vi "ROI entry-Event handler-Arb entry.vi"(8 "error in (no error)":errorcluster) -> (0 "error out":errorcluster)   [LabVIEW 2013]
uses:
  Typedefs/ROI ID Enum.ctl
  ROI Entry screen/Globals/gl_ROI Entry UI globals.vi
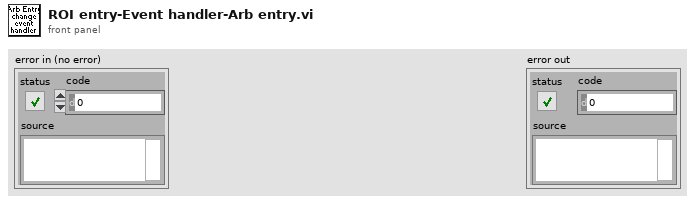
[diagram p1: front panel]
types:
  T1 = typedef "ROI entry screen ctrl refs cluster.ctl" = cluster{"Done button":refnum<vi>, "Imaging button":refnum<vi>, "Acquisition button":refnum<vi>, "POI dwell time (us)":refnum<vi>, "Scan dwell time per pixel (us)":refnum<vi>, "# of planes":refnum<vi>, "Zoom":refnum<vi>, "Equal size":refnum<vi>, "Channel":refnum<vi>, "Image Display":refnum<vi>, "Z-Plane Selector":refnum<vi>, "Number of lines left":refnum<vi>, "Z-stack folder path":refnum<vi>, "POI Density":refnum<vi>, "Arb Plane Entry":refnum<vi>, "Whole plane":refnum<vi>, "Clear Last":refnum<vi>, "Clear All":refnum<vi>, "Trial Length (sec)":refnum<vi>, "Palette Type":refnum<vi>, "Intensity slider":refnum<vi>, "# POI":refnum<vi>, "Max Z Proj":refnum<vi>, "Zplane ind":refnum<vi>, "Wavelength (nm)":refnum<vi>, "Number of Trials":refnum<vi>, "Funct stim.trig.enable":refnum<vi>, "Funct stim.trig.delay (s)":refnum<vi>, "Line Mode":refnum<vi>, "Step size (µm)":refnum<vi>, "ROI move mode":refnum<vi>, "Cool-down time (s)":refnum<vi>, "Enable cool-down time":refnum<vi>, "Motor Z ind. (um)":refnum<vi>, "AOL Z ind. (um)":refnum<vi>}
  T2 = typedef "ROI ID Enum.ctl" = enum16{"Point", "MiniScan", "Comp. MiniScan", "Rectangle", "Comp. volume", "Arb. plane point"}
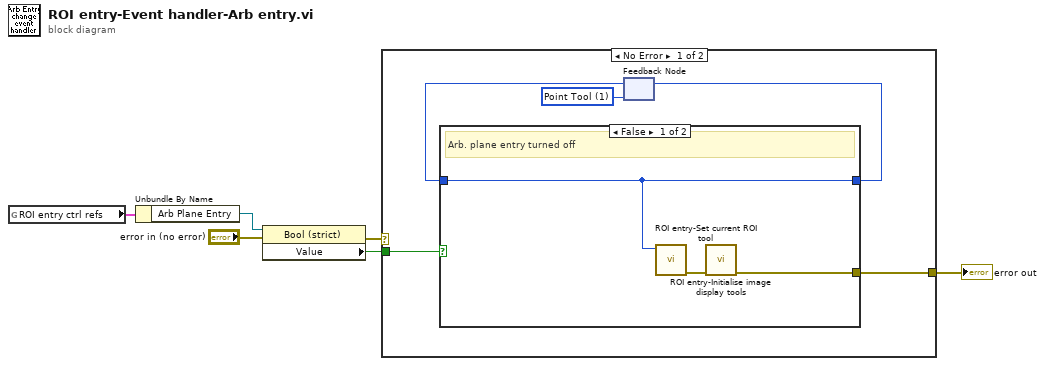
[diagram p0: block diagram]
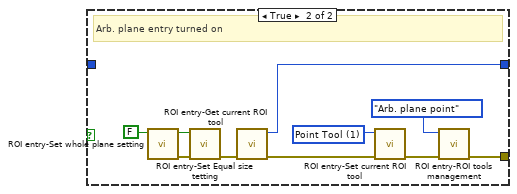
[diagram p2: hidden frame]
diagram:
  n1 = global read "gl_ROI Entry UI globals.vi" "ROI entry ctrl refs"() -> (w5:T1)
  n2 = Unbundle By Name(w5) -> ("Arb Plane Entry"=w6:refnum<vi>)
  n3 = property class="Bool (strict)"(reference=w6, error in="error in (no error)") -> (error out=w2:errorcluster, "Value"=w3:bool)  [unwired: 1 out]
  n4 = case shown="No Error" w2 {
    selector: w2 -> [_ w24]
    tunnel: [w9 w24] -> w4
    tunnel: w3 -> [w8 _]
    frame No Error {
      w11 = u32 1 items=["Zoom Tool"=8, "Selection Tool"=0, "Pan Tool"=9, "Point Tool"=1, "Line Tool"=2, "Rectangle Tool"=3, "Rotated Rectangle Tool"=12, "Polyline Tool"=10, "Polygon Tool"=5, "Freehand Tool"=11, "Closed Freehand Tool"=6, "Ellipse Tool"=4, "Annulus Tool"=7] ("Current ROI Tool")
      n5 = feedback #1(w11) -> (w10:u32)
      n6 = case shown="False" w8 {
        tunnel: [w14 w23] -> w7
        tunnel: w10 -> [w14 _]
        tunnel: [w12 w15] -> w9
        frame False {
          # "Arb. plane entry turned off"
          n7 = call "ROI entry-Set current ROI tool.vi"("Current ROI Tool"=w14) -> ("error out"=w13:errorcluster)  [unwired: 10 in]
          n8 = call "ROI entry-Initialise image display tools.vi"("error in (no error)"=w13) -> ("error out"=w12:errorcluster)  [unwired: 10 in]
        }
        frame True {
          w18 = FALSE ("\"Whole plane\" button's value")
          w21 = u32 1 items=["Zoom Tool"=8, "Selection Tool"=0, "Pan Tool"=9, "Point Tool"=1, "Line Tool"=2, "Rectangle Tool"=3, "Rotated Rectangle Tool"=12, "Polyline Tool"=10, "Polygon Tool"=5, "Freehand Tool"=11, "Closed Freehand Tool"=6, "Ellipse Tool"=4, "Annulus Tool"=7] ("Current ROI Tool")
          # "Arb. plane entry turned on"
          n9 = call "ROI entry-Set whole plane setting.vi"("\"Whole plane\" button's value"=w18) -> ("error out"=w20:errorcluster)  [unwired: 10 in]
          n10 = call "ROI entry-Set Equal size tetting.vi"("error in (no error)"=w20, "\"Equal size\" button's value"=w18) -> ("error out"=w19:errorcluster)  [unwired: 9 in]
          n11 = call "ROI entry-Get current ROI tool.vi"("error in (no error)"=w19) -> ("error out"=w22:errorcluster, "Current ROI Tool"=w23:u32)  [unwired: 9 in]
          n12 = call "ROI entry-Set current ROI tool.vi"("error in (no error)"=w22, "Current ROI Tool"=w21) -> ("error out"=w16:errorcluster)  [unwired: 9 in]
          n13 = call "ROI entry-ROI tools management.vi"("error in (no error)"=w16, "ROI Enum"=ROI_ID_Enum."Arb. plane point") -> ("error out"=w15:errorcluster)  [unwired: 9 in]
        }
      }
      n14 = feedback-in #1(w7) -> ()
    }
    frame Error {
    }
  }
  "error out" <- w4
